vi "Example.vi"() -> ()   [LabVIEW 2016]
panel:
  in  "Cluster":cluster{"Numeric":dbl}
  in  "Numeric":dbl
  in  "Tab Control":enum32{"Page 1", "Page 2"}(tab)
  in  "Knob":dbl(knob) scale=0.0..10.0
  in  "Boolean":bool
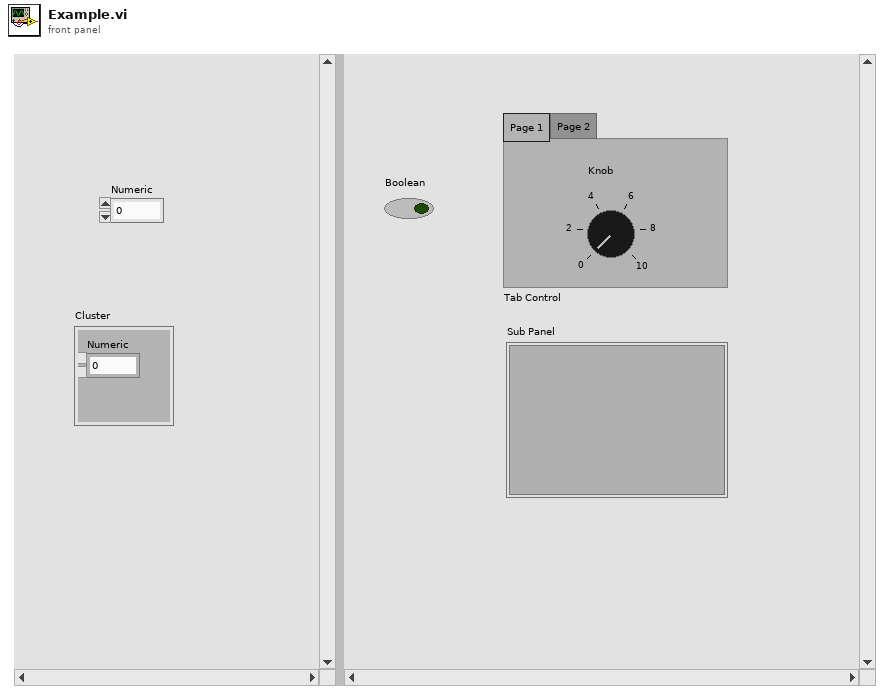
[diagram p1: front panel]
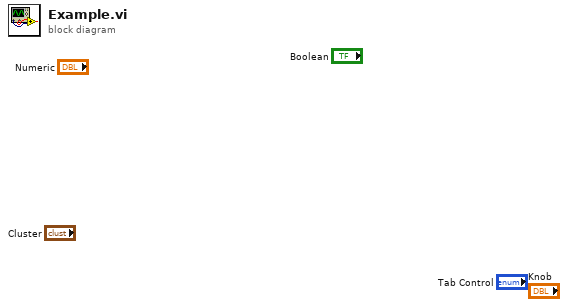
[diagram p0: block diagram]
diagram:
